vi "SR830.VI"(0 "GPIB address":string="8", 1 "input":T7 {"input" items=["A", "A-B", "I (1 M gain)", "I (100 M gain)"]}, 3 "channel 1":T3 {"output" items=["display", "X"]; "ratio" items=["none", "aux in 1", "aux in 2"]; "display" items=["X", "R", "X Noise", "Aux In 1", "Aux In 2"]}, 5 "sensitivity":T4={"sensitivity\n2nV/fA"=0, "dyn reserve\n(low noise:2)"=2, "ref. phase"=0.0, "automeasure"=FALSE} {"sensitivity\n2nV/fA" items=["2 nV/fA", "5 nV/fA", "10 nV/fA", "20 nV/fA", "50 nV/fA", "100 nV/fA", "200 nV/fA", "500 nV/fA", "1 µV /pA", "2 µV/pA", "5 µV/pA", "10 µV/pA", "20 µV/pA", "50 µV/pA", "100 µV/pA", "200 µV/pA", "500 µV/pA", "1 mV/nA", "2 mV/nA", "5 mV/nA", "10 mV/nA", "20 mV/nA", "50 mV/nA", "100 mV/nA", "200 mV/nA", "500 mV/nA", "1 V/µA"]; "dyn reserve\n(low noise:2)" scale=0.0..2.0 scale format="%.2f"; "ref. phase" format="%.2f"}, 7 "sync":T5 {"line filter\n(off:0)" items=["OFF", "line", "2 x line", "both"]}, 8 "reference":T8={"ref. source"=FALSE, "osc.harm# "=1, "osc. freq"=0.001, "osc. ampl."=0.004, "ref. trigger"=0} {"ref. trigger" items=["sine", "pos edge", "neg edge"]; "osc.harm#" min=1 max=19999; "osc. ampl." format="%.3f"; "osc. freq" format="%.3f"}, 9 "time constant":T6 {"slope (6 dB/oct)" items=["6 dB/oct", "12 dB/oct", "18 dB/oct", "24 dB/oct"]; "time constant\n(10 µs : 0)" items=["10 µs", "30 µs", "100 µs", "300 µs", "1 ms", "3 ms", "10 ms", "30 ms", "100 ms", "300 ms", "1 s", "3 s", "10 s", "30 s", "100 s", "300 s", "1 ks", "3 ks", "10 ks", "30 ks"]}, 10 "off. & exp.":T2 {"expand" items=["none", "x 10", "x 100"]; "offset" format="%.2f"; "off. & exp." items=["X", "Y", "R"]}, 11 "error in":T1, 14 "channel 2":T3={" display"=0, " ratio"=0, "output"=1} {"output" items=["display", "Y"]; "ratio" items=["none", "aux in 3", "aux in 4"]; "display" items=["Y", "@", "Y Noise", "Aux In 3", "Aux In 4"]}) -> (4 "CH 1 display":string, 6 "CH 2 display":string="\n", 15 "error out":T1)   [LabVIEW 2016]
doc: "This subVI implements all the basic functions of the SR830 DSP Lock-In Amplifier with the exception of setting the AUX OUTPUT voltages . This can be done in the SR830 AUX OUTPUT.vi"
panel:
  # "on\noff"
  # "on\noff"
  # "float\nground"
  # "AC\nDC"
  # "int\next"
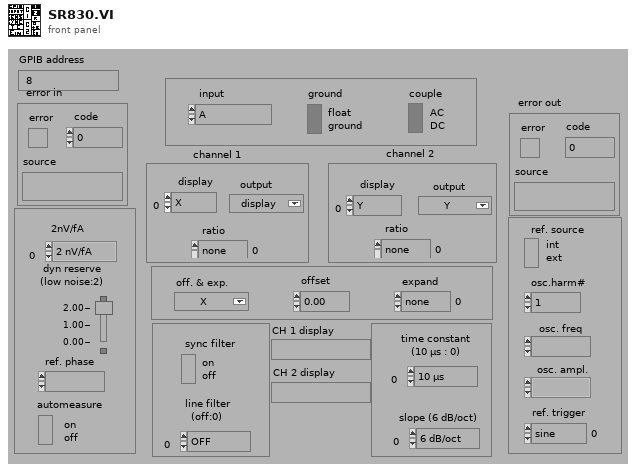
[diagram p1: front panel]
types:
  T1 = cluster{"error":bool, "code":i8, "source":string}
  T2 = cluster{"off. & exp.":u16, "offset":dbl, "expand":u16}
  T3 = cluster{" display":i32, " ratio":u16, "output":u16}
  T4 = cluster{"sensitivity\n2nV/fA":i32, "dyn reserve\n(low noise:2)":i16, "ref. phase":ext, "automeasure":bool}
  T5 = cluster{"sync filter":bool, "line filter\n(off:0)":i32}
  T6 = cluster{"time constant\n(10 µs : 0) ":i32, "slope (6 dB/oct)":i32}
  T7 = cluster{"input":u16, "ground":bool, "couple":bool}
  T8 = cluster{"ref. source":bool, "osc.harm# ":u16, "osc. freq":ext, "osc. ampl.":ext, "ref. trigger":u16}
  T9 = cluster{"error":bool, "code":i32, "source":string}
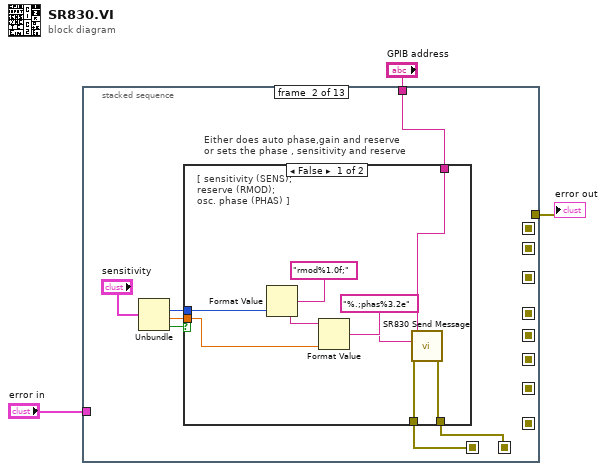
[diagram p0: block diagram]
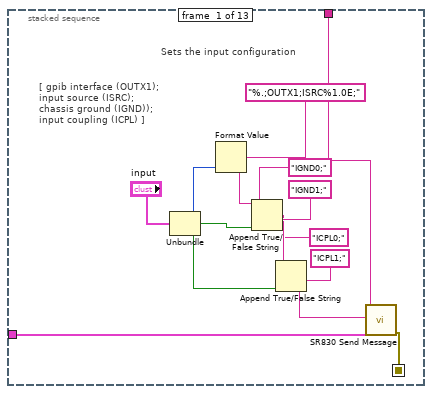
[diagram p2: hidden frame]
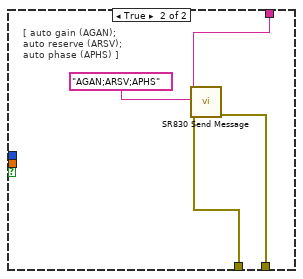
[diagram p3: hidden frame]
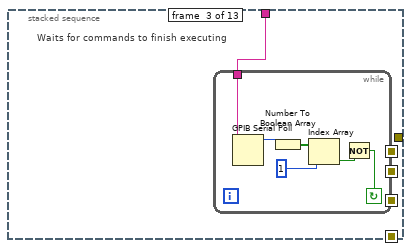
[diagram p4: hidden frame]
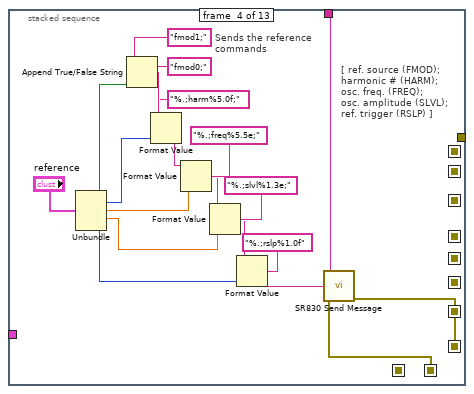
[diagram p5: hidden frame]
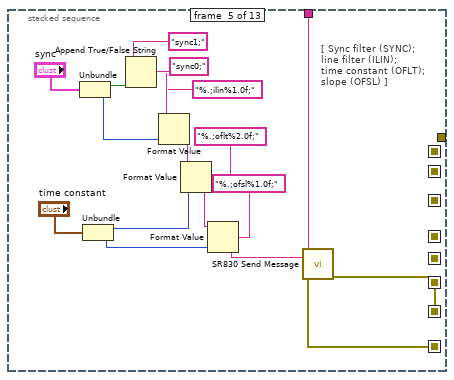
[diagram p6: hidden frame]
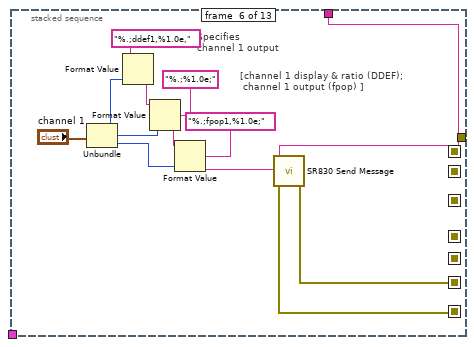
[diagram p7: hidden frame]
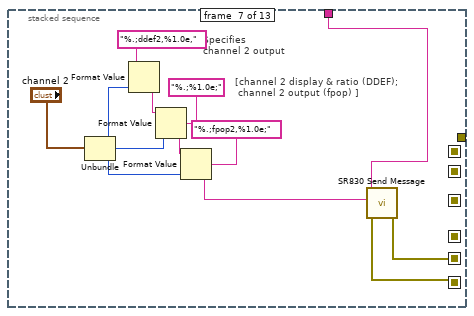
[diagram p8: hidden frame]
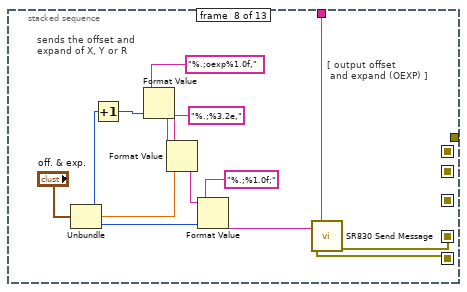
[diagram p9: hidden frame]
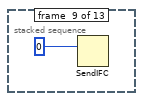
[diagram p10: hidden frame]
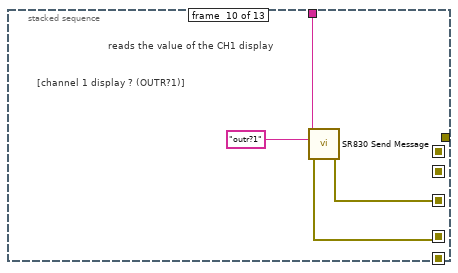
[diagram p11: hidden frame]
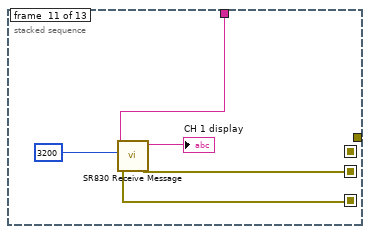
[diagram p12: hidden frame]
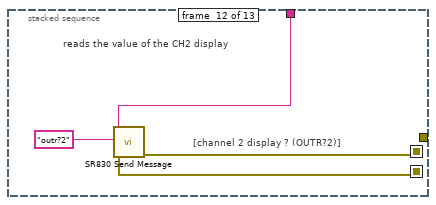
[diagram p13: hidden frame]
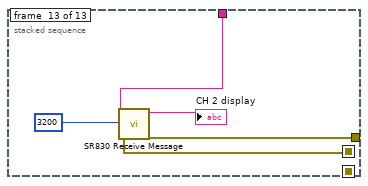
[diagram p14: hidden frame]
diagram:
  n1 = stacked-sequence {
    seq-local: [w4 _ _ _ _ _ _ _ _ _ _ _ _] -> [_ w20 _ _ _ _ _ _ _ _ _ _ _]
    seq-local: [_ w19 _ _ _ _ _ _ _ _ _ _ _] -> [_ _ _ w47 _ _ _ _ _ _ _ _ _]
    seq-local: [_ _ _ w46 _ _ _ _ _ _ _ _ _] -> [_ _ _ _ w67 _ _ _ _ _ _ _ _]
    seq-local: [_ _ _ _ w66 _ _ _ _ _ _ _ _] -> [_ _ _ _ _ w85 _ _ _ _ _ _ _]
    seq-local: [_ _ _ _ _ w84 _ _ _ _ _ _ _] -> [_ _ _ _ _ _ w98 _ _ _ _ _ _]
    seq-local: [_ _ _ _ _ _ w97 _ _ _ _ _ _] -> [_ _ _ _ _ _ _ w113 _ _ _ _ _]
    seq-local: [_ _ _ _ _ _ _ w112 _ _ _ _ _] -> [_ _ _ _ _ _ _ _ _ w125 _ _ _]
    seq-local: [_ _ _ _ _ _ _ _ _ w126 _ _ _] -> [_ _ _ _ _ _ _ _ _ _ w130 _ _]
    seq-local: [_ _ _ _ _ _ _ _ _ _ w129 _ _] -> [_ _ _ _ _ _ _ _ _ _ _ w135 _]
    seq-local: [_ _ _ _ _ _ _ _ _ _ _ w134 _] -> [_ _ _ _ _ _ _ _ _ _ _ _ w139]
    tunnel: "GPIB address" -> [w7 w24 w39 w49 w69 w87 w100 w115 _ w128 w133 w137 w142]
    tunnel: "error in" -> [w5 _ _ _ _ _ _ _ _ _ _ _ _]
    tunnel: [_ _ _ _ _ _ _ _ _ _ _ _ w138] -> w1
    frame #0 {
      # "[ gpib interface (OUTX1);\ninput source (ISRC);\nchassis ground (IGND));\ninput coupling (ICPL) ]"
      # "Sets the input configuration"
      n2 = Unbundle("input") -> ("input"=w10:u16, "ground"=w9:bool, "couple"=w8:bool)
      n3 = Format Value(format string="%.;OUTX1;ISRC%1.0E;", value (0)=w10) -> (output string=w17:string)  [unwired: 1 in]
      n4 = Append True/False String(1:w9, 2:"IGND1;", 3:"IGND0;", 4:w17) -> (0:w14:string)
      n5 = Append True/False String(1:w8, 2:"ICPL1;", 3:"ICPL0;", 4:w14) -> (0:w6:string)
      n6 = call "SR830 Send Message.vi"("address string"=w7, "write buffer"=w6, "error in"=w5) -> ("error out"=w4:T9)  [unwired: 4 in, 2 out]
    }
    frame #1 {
      # "Either does auto phase,gain and reserve\nor sets the phase , sensitivity and reserve"
      n7 = Unbundle("sensitivity") -> ("dyn reserve\n(low noise:2)"=w22:i16, "ref. phase"=w21:ext, "automeasure"=w23:bool)  [unwired: 1 out]
      n8 = case shown="False" w23 {
        tunnel: w24 -> [w29 w38]
        tunnel: w22 -> [w34 _]
        tunnel: w21 -> [w32 _]
        tunnel: w20 -> [w27 w36]
        tunnel: [w26 w35] -> w19
        frame False {
          # "[ sensitivity (SENS);\nreserve (RMOD);\nosc. phase (PHAS) ]"
          n9 = Format Value(format string="rmod%1.0f;", value (0)=w34) -> (output string=w31:string)  [unwired: 1 in]
          n10 = Format Value(string ("")=w31, format string="%.;phas%3.2e", value (0)=w32) -> (output string=w28:string)
          n11 = call "SR830 Send Message.vi"("address string"=w29, "write buffer"=w28, "error in"=w27) -> ("error out"=w26:T9)  [unwired: 4 in, 2 out]
        }
        frame True {
          # "[ auto gain (AGAN);\nauto reserve (ARSV);\nauto phase (APHS) ]"
          n12 = call "SR830 Send Message.vi"("address string"=w38, "write buffer"="AGAN;ARSV;APHS", "error in"=w36) -> ("error out"=w35:T9)  [unwired: 4 in, 2 out]
        }
      }
    }
    frame #2 {
      # "Waits for commands to finish executing"
      n13 = while {
        tunnel: w39 -> [w45]
        stop <- w40 continue-if-true
        n14 = GPIB Serial Poll(0:w45) -> (2:w44:i16)  [unwired: 1 in, 2 out]
        n15 = Number To Boolean Array(number=w44) -> (Boolean array=w43:bool[])
        n16 = Index Array(array=w43, index=1) -> (element=w41:bool)
        n17 = Not(x=w41) -> (.not. x?=w40:bool)
      }
    }
    frame #3 {
      # "[ ref. source (FMOD);\nharmonic # (HARM);\nosc. freq. (FREQ);\nosc. amplitude (SLVL);\nref. trigger (RSLP) ]"
      # "Sends the reference\ncommands"
      n18 = Unbundle("reference") -> ("ref. source"=w50:bool, "osc.harm#"=w62:u16, "osc. freq"=w59:ext, "osc. ampl."=w56:ext, "ref. trigger"=w51:u16)
      n19 = Append True/False String(1:w50, 2:"fmod0;", 3:"fmod1;") -> (0:w61:string)  [unwired: 1 in]
      n20 = Format Value(string ("")=w61, format string="%.;harm%5.0f;", value (0)=w62) -> (output string=w58:string)
      n21 = Format Value(string ("")=w58, format string="%.;freq%5.5e;", value (0)=w59) -> (output string=w55:string)
      n22 = Format Value(string ("")=w55, format string="%.;slvl%1.3e;", value (0)=w56) -> (output string=w53:string)
      n23 = Format Value(string ("")=w53, format string="%.;rslp%1.0f", value (0)=w51) -> (output string=w48:string)
      n24 = call "SR830 Send Message.vi"("address string"=w49, "write buffer"=w48, "error in"=w47) -> ("error out"=w46:T9)  [unwired: 4 in, 2 out]
    }
    frame #4 {
      # "[ Sync filter (SYNC);\nline filter (ILIN);\ntime constant (OFLT);\nslope (OFSL) ]"
      n25 = Unbundle("sync") -> ("sync filter"=w71:bool, "line filter\n(off:0)"=w70:i32)
      n26 = Unbundle("time constant") -> ("time constant\n(10 µs : 0)"=w77:i32, "slope (6 dB/oct)"=w76:i32)
      n27 = Append True/False String(1:w71, 2:"sync0;", 3:"sync1;") -> (0:w80:string)  [unwired: 1 in]
      n28 = Format Value(string ("")=w80, format string="%.;ilin%1.0f;", value (0)=w70) -> (output string=w74:string)
      n29 = Format Value(string ("")=w74, format string="%.;oflt%2.0f;", value (0)=w77) -> (output string=w73:string)
      n30 = Format Value(string ("")=w73, format string="%.;ofsl%1.0f;", value (0)=w76) -> (output string=w68:string)
      n31 = call "SR830 Send Message.vi"("address string"=w69, "write buffer"=w68, "error in"=w67) -> ("error out"=w66:T9)  [unwired: 4 in, 2 out]
    }
    frame #5 {
      # "[channel 1 display & ratio (DDEF);\n channel 1 output (fpop) ]"
      # "Specifies \nchannel 1 output"
      n32 = Unbundle("channel 1") -> ("display"=w90:i32, "ratio"=w89:u16, "output"=w88:u16)
      n33 = Format Value(format string="%.;ddef1,%1.0e,", value (0)=w90) -> (output string=w95:string)  [unwired: 1 in]
      n34 = Format Value(string ("")=w95, format string="%.;%1.0e;", value (0)=w89) -> (output string=w93:string)
      n35 = Format Value(string ("")=w93, format string="%.;fpop1,%1.0e;", value (0)=w88) -> (output string=w86:string)
      n36 = call "SR830 Send Message.vi"("address string"=w87, "write buffer"=w86, "error in"=w85) -> ("error out"=w84:T9)  [unwired: 4 in, 2 out]
    }
    frame #6 {
      # "[channel 2 display & ratio (DDEF);\n channel 2 output (fpop) ]"
      # "Specifies \nchannel 2 output"
      n37 = Unbundle("channel 2") -> ("display"=w103:i32, "ratio"=w102:u16, "output"=w101:u16)
      n38 = Format Value(format string="%.;ddef2,%1.0e,", value (0)=w103) -> (output string=w108:string)  [unwired: 1 in]
      n39 = Format Value(string ("")=w108, format string="%.;%1.0e;", value (0)=w102) -> (output string=w106:string)
      n40 = Format Value(string ("")=w106, format string="%.;fpop2,%1.0e;", value (0)=w101) -> (output string=w99:string)
      n41 = call "SR830 Send Message.vi"("address string"=w100, "write buffer"=w99, "error in"=w98) -> ("error out"=w97:T9)  [unwired: 4 in, 2 out]
    }
    frame #7 {
      # "[ output offset\n and expand (OEXP) ]"
      # "sends the offset and\nexpand of X, Y or R"
      n42 = Unbundle("off. & exp.") -> ("off. & exp."=w122:u16, "offset"=w111:dbl, "expand"=w117:u16)
      n43 = Increment(x=w122) -> (x+1=w110:u16)
      n44 = Format Value(format string="%.;oexp%1.0f,", value (0)=w110) -> (output string=w120:string)  [unwired: 1 in]
      n45 = Format Value(string ("")=w120, format string="%.;%3.2e,", value (0)=w111) -> (output string=w118:string)
      n46 = Format Value(string ("")=w118, format string="%.;%1.0f;", value (0)=w117) -> (output string=w114:string)
      n47 = call "SR830 Send Message.vi"("address string"=w115, "write buffer"=w114, "error in"=w113) -> ("error out"=w112:T9)  [unwired: 4 in, 2 out]
    }
    frame #8 {
      n48 = SendIFC(3:0) -> ()  [unwired: 1 in, 2 out]
    }
    frame #9 {
      # "[channel 1 display ? (OUTR?1)]"
      # "reads the value of the CH1 display"
      n49 = call "SR830 Send Message.vi"("address string"=w128, "write buffer"="outr?1", "error in"=w125) -> ("error out"=w126:T9)  [unwired: 4 in, 2 out]
    }
    frame #10 {
      n50 = call "SR830 Receive Message.vi"("address string"=w133, "byte count"=3200, "error in"=w130) -> ("read buffer"=→"CH 1 display":string, "error out"=w129:T9)  [unwired: 4 in, 1 out]
    }
    frame #11 {
      # "[channel 2 display ? (OUTR?2)]"
      # "reads the value of the CH2 display"
      n51 = call "SR830 Send Message.vi"("address string"=w137, "write buffer"="outr?2", "error in"=w135) -> ("error out"=w134:T9)  [unwired: 4 in, 2 out]
    }
    frame #12 {
      n52 = call "SR830 Receive Message.vi"("address string"=w142, "byte count"=3200, "error in"=w139) -> ("read buffer"=→"CH 2 display":string, "error out"=w138:T9)  [unwired: 4 in, 1 out]
    }
  }
  "error out" <- w1
